vi "Scalar Bitpacked.vi"(8 "error in (no error)":errorcluster, 11 "Node Ptr":T1 format="%.0x") -> (0 "error out":errorcluster)   [LabVIEW 2016, in "FPGA Addon System Explorer.lvlib"]
uses:
  FPGA Addon System Explorer.lvlib
  <vilib>/NI Veristand/Custom Device API/Custom Device Item Ref.ctl
  Shared/FG Action.ctl
  <vilib>/NI Veristand/Custom Device API/Custom Device Channel.ctl
  <vilib>/NI Veristand/Custom Device API/Custom Device Channel Type.ctl
  Shared/get fpga resource values for cd group.vi
  Shared/Constants.vi
  <vilib>/NI Veristand/Custom Device API/Get Item Property (U32).vi
  <vilib>/NI Veristand/Custom Device API/NI VeriStand - Set Item Property.vi
  <vilib>/NI Veristand/Custom Device API/Set Item Property (U32).vi
  <vilib>/NI Veristand/Custom Device API/Get Item Property (String).vi
  FPGA-Resource-Manager-APIs/Source/find Relative VS Ref.vi
  FPGA-Resource-Manager-APIs/Source/get fgpa resources.vi
  SubVIs/convert RegisterMap to FPGA Scalar.vi
  <vilib>/NI Veristand/Custom Device Tools/Custom Device Utility Library/NI VeriStand - Search for All Items by GUID.vi
  <vilib>/NI VeriStand/Custom Device API/Custom Device API.lvlib
  Shared/FPGA Addon Shared.lvlib
  <vilib>/NI VeriStand/Custom Device Tools/Custom Device Utility Library/Custom Device Utility Library.lvlib
panel:
  out "Original Name":string
  in  "SHDocVw.IWebBrowser":refnum<k7>(container)
  in  "Reset":bool
  in  "Apply":bool
  in  "Number of Channels":u8
  in  "Header 2":cluster{"Section Name":string}={"Section Name"="Custom Device Item Settings"}
  in  "Header":cluster{"Section Name":string}={"Section Name"="Custom Device Item Settings"}
  in  "Description":string
  in  "Name":string
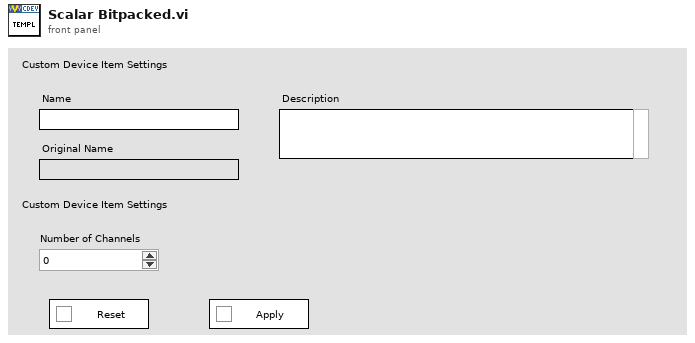
[diagram p1: front panel]
types:
  T1 = typedef "Custom Device API.lvlib/Custom Device Item Ref.ctl" = u64
  T2 = typedef "FPGA Addon Shared.lvlib/FG Action.ctl" = enum8{"GET", "SET"}
  T3 = typedef "FPGA Addon Shared.lvlib/Scalar Settings.ctl" = cluster{"Number of Channels":u8}
  T4 = typedef "FPGA Addon Shared.lvlib/Register Information.ctl" = cluster{"Name":string, "Data Type":T5, "Default Value":variant}
  T5 = typedef "FPGA Addon Shared.lvlib/Data Type.ctl" = enum8{"<Null>", "I8", "I16", "I32", "I64", "U8", "U16", "U32", "U64", "SGL", "Boolean", "Analog PWM In Settings", "Analog PWM In", "Digital PWM In Settings", "Digital PWM In", "Digital PWM Out", "Sine Out", "FXP+/-24.5", "FXP+/-16.5", "FXP+/-32.8", "FXP+/-64.32", "FXP+/-16.7", "FXP+/-20.5"}
  T6 = typedef "Custom Device API.lvlib/Custom Device Item Info.ctl" = cluster{"Name":string, "Is Channel":bool, "GUID":string, "Is Waveform":bool}
  T7 = typedef "Custom Device API.lvlib/Custom Device Channel.ctl" = cluster{"Type":T8, "Units":string, "Default Value":dbl, "Faultable":bool, "Scalable":bool}
  T8 = typedef "Custom Device API.lvlib/Custom Device Channel Type.ctl" = enum16{"Input", "Output"}
  T9 = typedef "Custom Device API.lvlib/Custom Device Commands.ctl" = enum16{"Default", "Item renamed", "Shutdown", "Dynamic button pressed"}
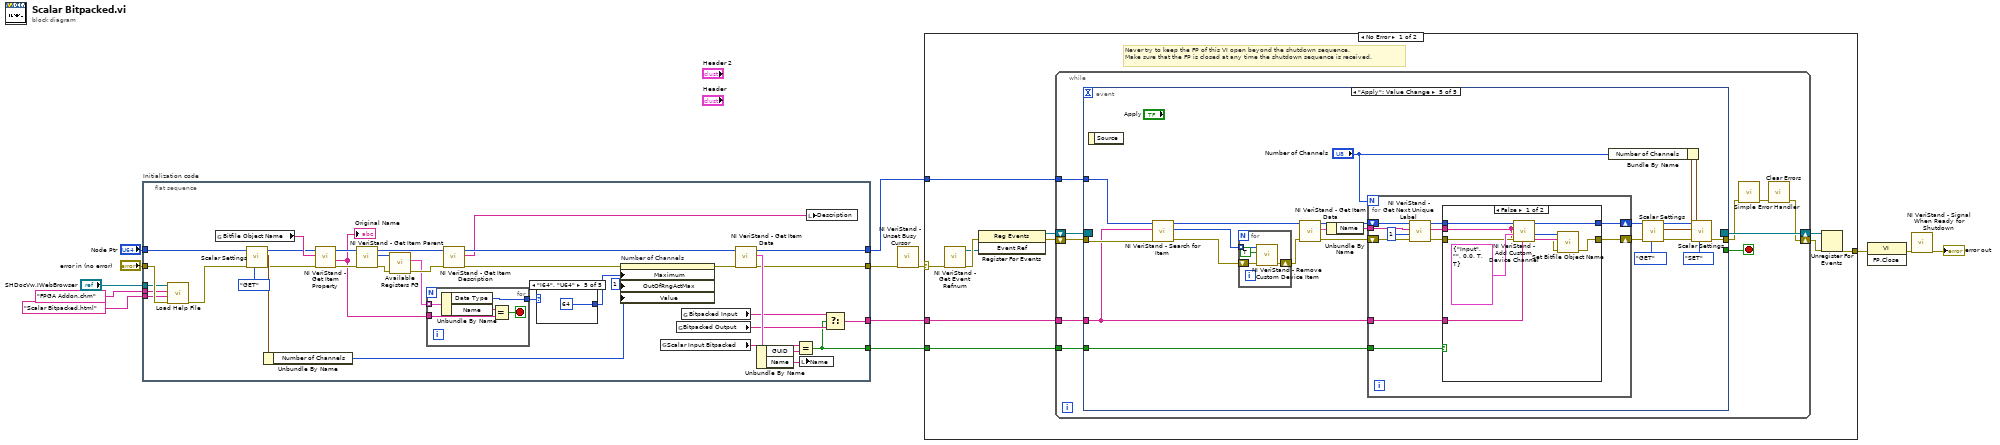
[diagram p0: block diagram]
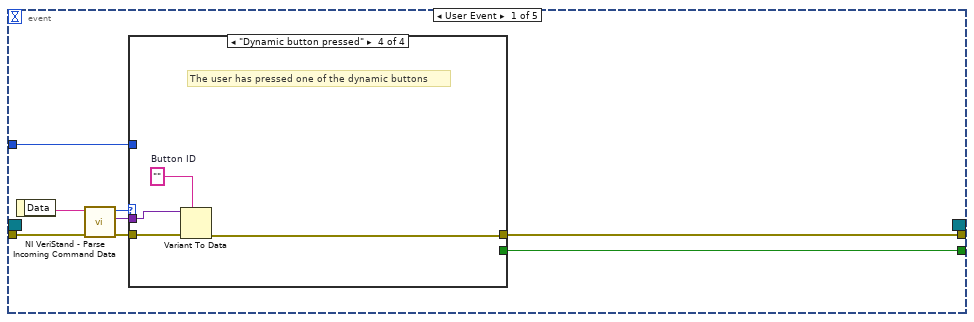
[diagram p2: hidden frame]
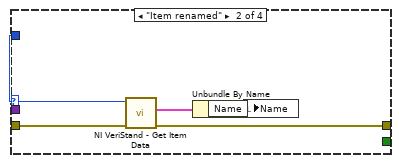
[diagram p4: hidden frame]
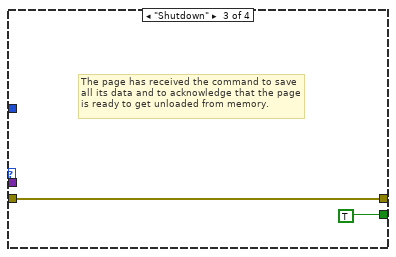
[diagram p5: hidden frame]
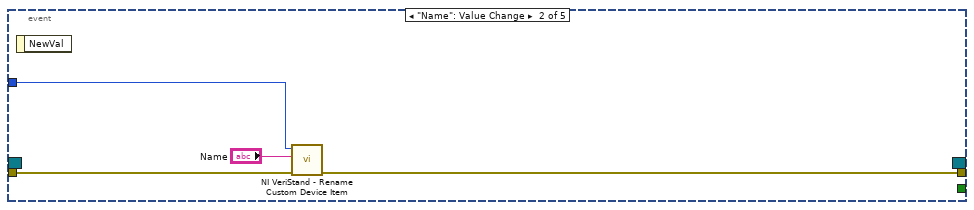
[diagram p6: hidden frame]
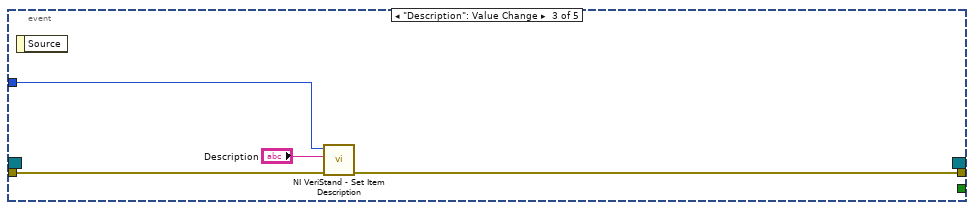
[diagram p7: hidden frame]
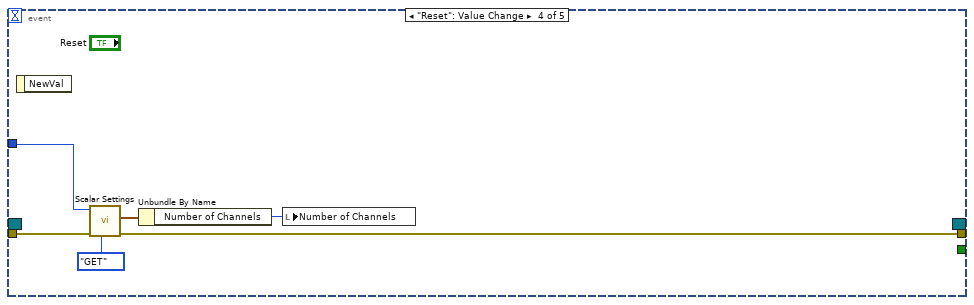
[diagram p8: hidden frame]
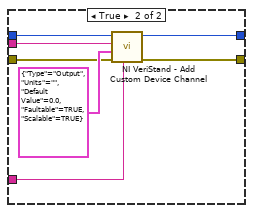
[diagram p9: hidden frame]
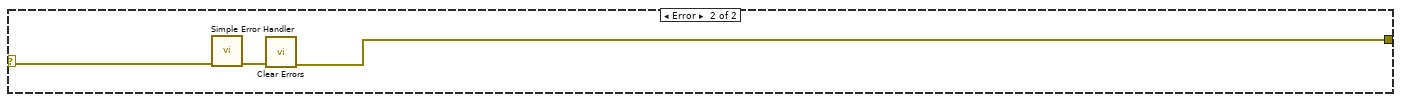
[diagram p10: hidden frame]
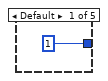
[diagram p11: hidden frame]
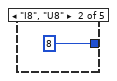
[diagram p12: hidden frame]
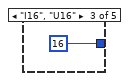
[diagram p13: hidden frame]
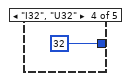
[diagram p14: hidden frame]
diagram:
  n1 = flat-sequence "Initialization code" {
    tunnel: "error in (no error)" -> [w19]
    tunnel: "Node Ptr" -> [w27]
    tunnel: [w46] -> w10
    tunnel: [w47] -> w8
    tunnel: [w42] -> w5
    tunnel: [w41] -> w4
    tunnel: "SHDocVw.IWebBrowser" -> [w17]
    tunnel: "FPGA Addon.chm" ("Main CHM File") -> [w16]
    tunnel: "Scalar Bitpacked.html" ("HTML File") -> [w15]
    frame #0 {
      n2 = call "Load Help File.vi"("error in (no error)"=w19, "HTML File"=w15, "Main CHM File"=w16, "SHDocVw.IWebBrowser2"=w17) -> ("error out"=w18:errorcluster)  [unwired: 7 in]
      n3 = global read "Constants.vi" "Bitfile Object Name"() -> (w32:string)
      n4 = call "Scalar Settings.vi"("Action"=FG_Action."GET", "error in (no error)"=w18, "Item Ref"=w27) -> ("error out"=w26:errorcluster, "Scalar Settings"=w38:T3, "Item Ref out"=w25:T1)  [unwired: 6 in]
      n5 = Unbundle By Name(w38) -> ("Number of Channels"=w30:u8)
      n6 = call-poly <vilib>:"NI VeriStand - Get Item Property.vi"("error in (no error)"=w26, "Property Name"=w32, "Item Ref in"=w25) -> ("error out"=w23:errorcluster, "Value"=w14:string, "Item Ref out"=w24:T1)  [unwired: 5 in, 1 out]
      "Original Name" <- w14
      n7 = call <vilib>:"NI VeriStand - Get Item Parent.vi"("error in (no error)"=w23, "Item Ref in"=w24) -> ("error out"=w35:errorcluster, "Parent Ref"=w36:T1, "Item Ref out"=w37:T1)  [unwired: 6 in, 1 out]
      n8 = call "Available Registers FG.vi"("error in (no error)"=w35, "Item Ref"=w36) -> ("error out"=w34:errorcluster, "Available Registers"=w33:T4[])  [unwired: 7 in, 1 out]
      n9 = for {
        tunnel: w33 -> [w60] mode=indexing
        tunnel: w14 -> [w58]
        tunnel: [w56] -> w29
        stop <- w57 stop-if-true
        n10 = Unbundle By Name(w60) -> ("Data Type"=w56:T5, "Name"=w59:string)
        n11 = Equal?(x=w59, y=w58) -> (x = y?=w57:bool)
      }
      n12 = call <vilib>:"NI VeriStand - Get Item Description.vi"("error in (no error)"=w34, "Item Ref in"=w37) -> ("error out"=w22:errorcluster, "Description"=w49:string, "Item Ref out"=w50:T1)  [unwired: 7 out]
      n13 = case shown="\"I64\", \"U64\"" w29 {
        tunnel: [1 8 16 32 64] -> w28
        frame Default {
        }
        frame "I8", "U8" {
        }
        frame "I16", "U16" {
        }
        frame "I32", "U32" {
        }
        frame "I64", "U64" {
        }
      }
      n14 = property on="Number of Channels" class="DigNum (strict)"(error in=w22, "Maximum"=w28, "OutOfRngActMax"=u8 1 ("Response to Value Outside Limits:Maximum"), "Value"=w30) -> (error out=w21:errorcluster)  [unwired: 1 in, 1 out]
      n15 = global read "Constants.vi" "Scalar Input Bitpacked"() -> (w45:string)
      n16 = global read "Constants.vi" "Bitpacked Output"() -> (w44:string)
      n17 = global read "Constants.vi" "Bitpacked Input"() -> (w43:string)
      n18 = call <vilib>:"NI VeriStand - Get Item Data.vi"("error in (no error)"=w21, "Item Ref in"=w50) -> ("error out"=w46:errorcluster, "Item Info"=w48:T6, "Item Ref out"=w47:T1)  [unwired: 7 out]
      n19 = Unbundle By Name(w48) -> ("GUID"=w40:string, "Name"=w20:string)
      n20 = Equal?(x=w45, y=w40) -> (x = y?=w42:bool)
      n21 = local write "Name"(w20) -> ()
      n22 = local write "Description"(w49) -> ()
      n23 = Select(t=w43, s=w42, f=w44) -> (s? t:f=w41:string)
    }
  }
  n24 = call <vilib>:"NI VeriStand - Unset Busy Cursor.vi"("error in (no error)"=w10) -> ("error out"=w9:errorcluster)  [unwired: 10 out]
  n25 = case shown="No Error" w9 {
    selector: w9 -> [w63 w171]
    tunnel: [w68 w169] -> w13
    tunnel: w8 -> [w64 _]
    tunnel: w5 -> [w62 _]
    tunnel: w4 -> [w61 _]
    frame No Error {
      # "Never try to keep the FP of this VI open beyond the shutdown sequence.\nMake sure that the FP is closed at any time the shutdown sequence is received."
      n26 = call <vilib>:"NI VeriStand - Get Event Refnum.vi"("error in (no error)"=w63) -> ("error out"=w71:errorcluster, "Event Ref"=w67:refnum<user-event>)  [unwired: 9 out]
      n27 = register-events(error in=w71, w67) -> (reference out=w65:refnum<event-registration>, error out=w66:errorcluster)  [unwired: 1 in]
      n28 = while {
        tunnel: w64 -> [w77]
        shift-right: [w74] -> w69
        shift-left: w66 -> [w80]
        shift-right: [w81] -> w70
        shift-left: w65 -> [w79]
        tunnel: w62 -> [w73]
        tunnel: w61 -> [w72]
        stop <- w78 stop-if-true
        n29 = event shown="[4] \"Apply\": Value Change" {
          selector: w79 -> [_ _ _ _ _]
          dyn-events: [_ _ _ _ _] -> w81
          timeout: _ -> [_ _ _ _ _]
          tunnel: w80 -> [w89 w105 w108 w115 w123]
          tunnel: [w85 _ _ _ _] -> w78
          tunnel: [w84 w104 w107 w111 w129] -> w76
          tunnel: w77 -> [w83 w103 w109 w113 w124]
          tunnel: w73 -> [_ _ _ _ w125]
          tunnel: w72 -> [_ _ _ _ w120]
          event User Event {
            n30 = event-data() -> ("Data"=w88:string)  [unwired: 1 out]
            n31 = call <vilib>:"NI VeriStand - Parse Incoming Command Data.vi"("error in (no error)"=w89, "Incoming data"=w88) -> ("error out"=w87:errorcluster, "Outgoing data"=w82:variant, "Action"=w86:T9)  [unwired: 7 out]
            n32 = case shown="\"Dynamic button pressed\"" w86 {
              tunnel: w87 -> [w90 w95 w96 w101]
              tunnel: [_ _ TRUE _] -> w85
              tunnel: [w90 w92 w96 w98] -> w84
              tunnel: w83 -> [_ w94 _ _]
              tunnel: w82 -> [_ _ _ w100]
              frame "Default", Default {
              }
              frame "Item renamed" {
                n33 = call <vilib>:"NI VeriStand - Get Item Data.vi"("error in (no error)"=w95, "Item Ref in"=w94) -> ("error out"=w92:errorcluster, "Item Info"=w93:T6)  [unwired: 8 out]
                n34 = Unbundle By Name(w93) -> ("Name"=w91:string)
                n35 = local write "Name"(w91) -> ()
              }
              frame "Shutdown" {
                # "The page has received the command to save all its data and to acknowledge that the page is ready to get unloaded from memory."
              }
              frame "Dynamic button pressed" {
                w99 = ""  # Button ID
                # "The user has pressed one of the dynamic buttons"
                n36 = Variant To Data(error in=w101, type=w99, Variant=w100) -> (error out=w98:errorcluster)  [unwired: 1 out]
              }
            }
          }
          event "Name": Value Change {
            n37 = event-data() -> ()  [unwired: 2 out]
            n38 = call <vilib>:"NI VeriStand - Rename Custom Device Item.vi"("error in (no error)"=w105, "New Name"="Name", "Item Ref in"=w103) -> ("error out"=w104:errorcluster)  [unwired: 1 in, 7 out]
          }
          event "Description": Value Change {
            n39 = event-data() -> ()  [unwired: 2 out]
            n40 = call <vilib>:"NI VeriStand - Set Item Description.vi"("error in (no error)"=w108, "Description"="Description", "Item Ref in"=w109) -> ("error out"=w107:errorcluster)  [unwired: 8 out]
          }
          event "Reset": Value Change {
            n41 = event-data() -> ()  [unwired: 2 out]
            n42 = call "Scalar Settings.vi"("Action"=FG_Action."GET", "error in (no error)"=w115, "Item Ref"=w113) -> ("error out"=w111:errorcluster, "Scalar Settings"=w112:T3)  [unwired: 6 in, 1 out]
            n43 = Unbundle By Name(w112) -> ("Number of Channels"=w110:u8)
            n44 = local write "Number of Channels"(w110) -> ()
          }
          event "Apply": Value Change {
            n45 = event-data() -> ()  [unwired: 2 out]
            n46 = call-poly <vilib>:"NI VeriStand - Search for Item.vi"("error in"=w123, "Item GUID"=w120, "Section Ref in"=w124) -> ("error out"=w121:errorcluster, "Item Refs"=w119:T1[], "Section Ref out"=w122:T1)  [unwired: 5 in, 1 out]
            n47 = for {
              shift-right: [w140] -> w136
              shift-left: w121 -> [w141]
              tunnel: w119 -> [w138] mode=indexing
              n48 = call <vilib>:"NI VeriStand - Remove Custom Device Item.vi"("error in (no error)"=w141, "Force Delete (F)"=TRUE, "Item Ref in"=w138) -> ("error out"=w140:errorcluster)  [unwired: 7 in, 1 out]
            }
            n49 = call <vilib>:"NI VeriStand - Get Item Data.vi"("error in (no error)"=w136, "Item Ref in"=w122) -> ("error out"=w118:errorcluster, "Item Info"=w135:T6, "Item Ref out"=w116:T1)  [unwired: 7 out]
            n50 = Unbundle By Name(w135) -> ("Name"=w117:string)
            n51 = for {
              N: "Number of Channels" -> [_]
              tunnel: w117 -> [w146]
              shift-right: [w152] -> w134
              shift-left: w118 -> [w148]
              shift-right: [w144] -> w133
              shift-left: w116 -> [w147]
              tunnel: w120 -> [w143]
              tunnel: w125 -> [w142]
              n52 = call <vilib>:"NI VeriStand - Get Next Unique Label.vi"("error in (no error)"=w148, "Start Value (1)"=1, "Label"=w146, "Parent Ref in"=w147) -> ("error out"=w151:errorcluster, "Label out"=w149:string, "Parent Ref dup"=w150:T1)  [unwired: 4 in, 1 out]
              n53 = case shown="False" w142 {
                tunnel: [w153 w164] -> w152
                tunnel: w151 -> [w159 w165]
                tunnel: w150 -> [w160 w167]
                tunnel: w149 -> [w155 w166]
                tunnel: [w158 w163] -> w144
                tunnel: w143 -> [w157 w162]
                frame False {
                  n54 = call <vilib>:"NI VeriStand - Add Custom Device Channel.vi"("GUID (Default Channel)"=w157, "error in (no error)"=w159, "Channel"=T7 {"Type"=enum."Input", "Units"="", "Default Value"=0.0, "Faultable"=TRUE, "Scalable"=TRUE}, "Channel Name"=w155, "Parent Ref in"=w160) -> ("error out"=w154:errorcluster, "Channel Ref"=w156:T1, "Parent Ref out"=w158:T1)  [unwired: 3 in, 1 out]
                  n55 = call "Set Bitfile Object Name.vi"("error in (no error)"=w154, "Name"=w155, "Channel Ref"=w156) -> ("error out"=w153:errorcluster)  [unwired: 8 in]
                }
                frame True {
                  n56 = call <vilib>:"NI VeriStand - Add Custom Device Channel.vi"("GUID (Default Channel)"=w162, "error in (no error)"=w165, "Channel"=T7 {"Type"=enum."Output", "Units"="", "Default Value"=0.0, "Faultable"=TRUE, "Scalable"=TRUE}, "Channel Name"=w166, "Parent Ref in"=w167) -> ("error out"=w164:errorcluster, "Parent Ref out"=w163:T1)  [unwired: 3 in, 2 out]
                }
              }
            }
            n57 = call "Scalar Settings.vi"("Action"=FG_Action."GET", "error in (no error)"=w134, "Item Ref"=w133) -> ("error out"=w130:errorcluster, "Scalar Settings"=w128:T3, "Item Ref out"=w131:T1)  [unwired: 6 in]
            n58 = Bundle By Name(cluster=w128, "Number of Channels"="Number of Channels") -> (w127:T3)
            n59 = call "Scalar Settings.vi"("Action"=FG_Action."SET", "error in (no error)"=w130, "Scalar Settings"=w127, "Item Ref"=w131) -> ("error out"=w129:errorcluster)  [unwired: 5 in, 2 out]
          }
        }
        n60 = call <vilib>:"Simple Error Handler.vi"("error in (no error)"=w76) -> ("error out"=w75:errorcluster)  [unwired: 1 in, 7 out]
        n61 = call <vilib>:"Clear Errors.vi"("error in (no error)"=w75) -> ("error out"=w74:errorcluster)  [unwired: 1 in, 5 out]
      }
      n62 = Unregister For Events(event registration refnum=w70, error in=w69) -> (error out=w68:errorcluster)
    }
    frame Error {
      n63 = call <vilib>:"Simple Error Handler.vi"("error in (no error)"=w171) -> ("error out"=w170:errorcluster)  [unwired: 1 in, 7 out]
      n64 = call <vilib>:"Clear Errors.vi"("error in (no error)"=w170) -> ("error out"=w169:errorcluster)  [unwired: 1 in, 5 out]
    }
  }
  n65 = invoke class="VI" method="FP.Close"(error in=w13) -> (error out=w12:errorcluster)  [unwired: 2 in, 2 out]
  n66 = call <vilib>:"NI VeriStand - Signal When Ready for Shutdown.vi"("error in (no error)"=w12) -> ("error out"=→"error out":errorcluster)  [unwired: 10 out]
